vi "Read.vi"(11 "Load Result Value in":refnum<class "Load Result Value.lvclass">) -> (2 "Load Result":T1)   [LabVIEW 2020, in "VolatusSeq.lvlib" / "Load Result Value.lvclass"]
uses:
  Load Result Value.lvclass
  Load Result Value.lvclass/Load Result Value.ctl
  Load Result.ctl
  VolatusSeq.lvlib
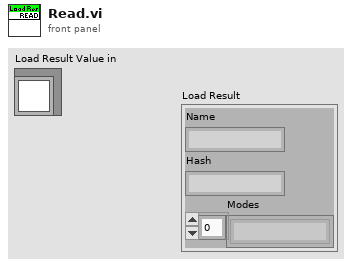
[diagram p1: front panel]
types:
  T1 = typedef "VolatusSeq.lvlib/Load Result.ctl" = cluster{"Name":string, "Hash":string, "Modes":string[]}
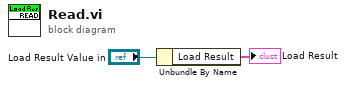
[diagram p0: block diagram]
diagram:
  n1 = Unbundle By Name("Load Result Value in") -> ("Load Result"=→"Load Result":T1)
